vi "TestExec.Get Sequence List.vi"(8 "error in":errorcluster, 10 "Working Config File":path, 11 "Working Dir":path) -> (0 "error out":errorcluster, 1 "Default Index":i32, 2 "Sequences Info":T1[](array[typedef]), 3 "Seq Names":string[](array[string]), 4 "Repeat Delay":dbl, 6 "AutoRepeat":bool)   [LabVIEW 2018]
uses:
  Controls and Type Defs/TestExec.Sequence Info.ctl
  <vilib>/Utility/config.llb/Read Key (String).vi
  <vilib>/Utility/config.llb/Read Key (Boolean).vi
  <vilib>/Utility/config.llb/Read Key (Double).vi
  <vilib>/Utility/config.llb/NI_LVConfig.lvlib
  <vilib>/KATE/Files/File Utils.lvlib
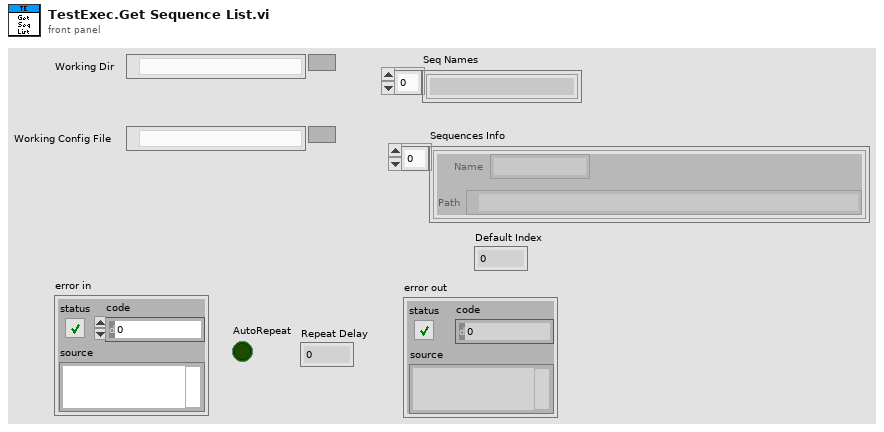
[diagram p1: front panel]
types:
  T1 = typedef "TestExec.Sequence Info.ctl" = cluster{"Name":string, "Path":path}
  T2 = typedef "NI_LVConfig.lvlib/Config Data RefNum.ctl" = refnum<k1>
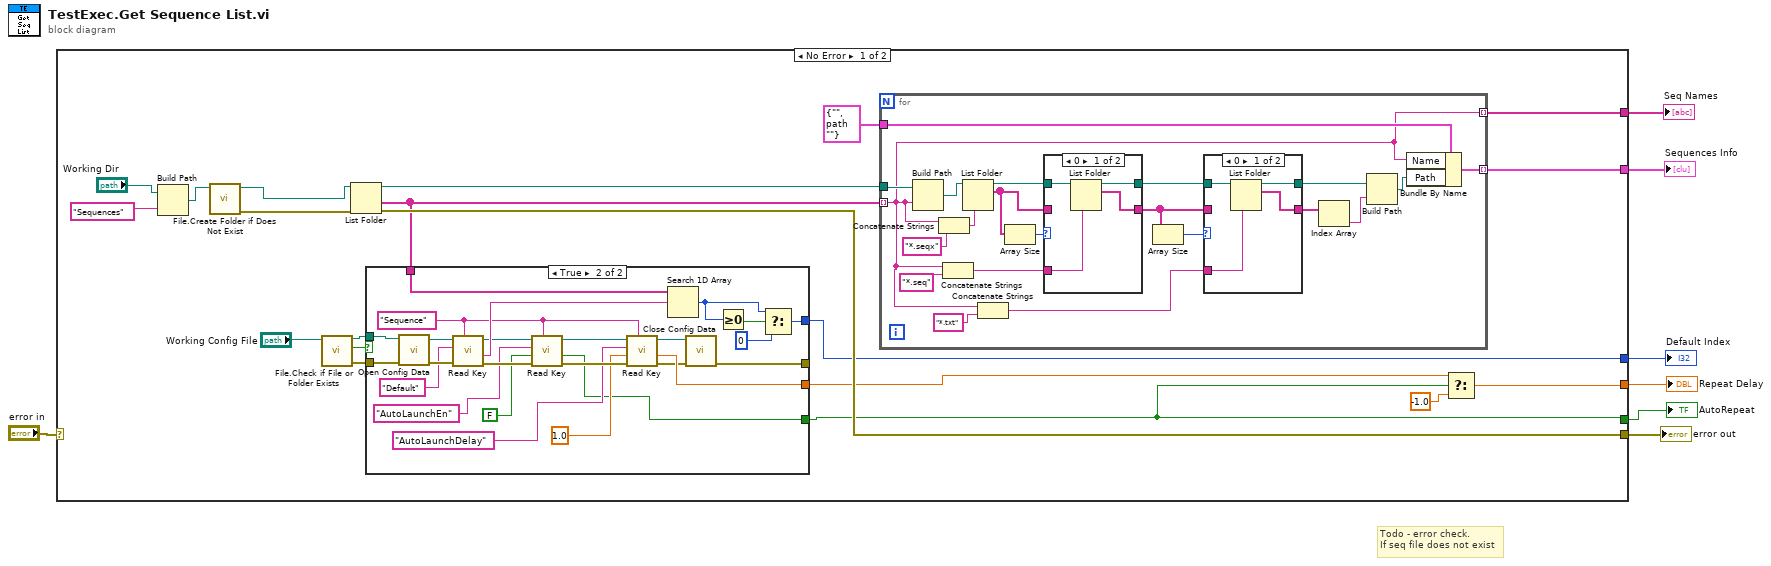
[diagram p0: block diagram]
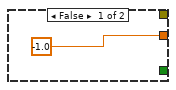
[diagram p2: hidden frame]
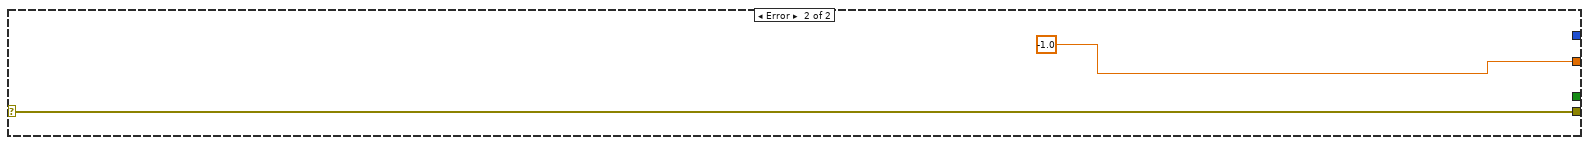
[diagram p5: hidden frame]
diagram:
  # "Todo - error check.\nIf seq file does not exist"
  n1 = case shown="No Error" "error in" {
    selector: "error in" -> [_ w88]
    tunnel: [w24 _] -> w7
    tunnel: [w23 w88] -> w5
    tunnel: [w22 _] -> w4
    tunnel: [w17 _] -> w3
    tunnel: [w12 -1.0] -> w2
    tunnel: [w9 _] -> w1
    frame No Error {
      n2 = Build Path(base path="Working Dir", name or relative path="Sequences" ("section")) -> (appended path=w16:path)
      n3 = call <vilib>:"File.Create Folder if Does Not Exist.vi"("Path"=w16) -> ("error out"=w14:errorcluster, "Dup Path"=w15:path)  [unwired: 8 in, 1 out]
      n4 = call <vilib>:"File.Check if File or Folder Exists.vi"("Path"="Working Config File") -> ("error out"=w18:errorcluster, "Exists"=w20:bool, "Dup Path"=w19:path)  [unwired: 6 in, 2 out]
      n5 = List Folder(path=w15, error in=w14) -> (path out=w26:path, folder names=w21:string[], error out=w23:errorcluster)  [unwired: 2 in, 1 out]
      n6 = case shown="True" w20 {
        tunnel: w21 -> [_ w50]
        tunnel: w19 -> [_ w49]
        tunnel: w18 -> [_ w48]
        tunnel: [_ w47] -> _
        tunnel: [_ w43] -> w17
        tunnel: [-1.0 w34] -> w11
        tunnel: [_ w29] -> w9
        frame False {
        }
        frame True {
          w35 = "Sequence"
          n7 = call <vilib>:"Open Config Data.vi"("error in (no error)"=w48, "configuration file path"=w49) -> ("error out"=w53:errorcluster, "refnum"=w52:T2)  [unwired: 7 in, 1 out]
          n8 = call-poly <vilib>:"Read Key.vi"("section"=w35, "error in (no error)"=w53, "key"="Default", "refnum"=w52) -> ("error out"=w42:errorcluster, "value"=w41:string, "refnum out"=w40:T2)  [unwired: 4 in, 1 out]
          n9 = call-poly <vilib>:"Read Key.vi"("section"=w35, "error in (no error)"=w42, "default value"=FALSE, "key"="AutoLaunchEn", "refnum"=w40) -> ("error out"=w33:errorcluster, "value"=w29:bool, "refnum out"=w37:T2)  [unwired: 3 in, 1 out]
          n10 = call-poly <vilib>:"Read Key.vi"("section"=w35, "error in (no error)"=w33, "default value"=1.0, "key"="AutoLaunchDelay", "refnum"=w37) -> ("error out"=w32:errorcluster, "value"=w34:dbl, "refnum out"=w36:T2)  [unwired: 3 in, 1 out]
          n11 = Search 1D Array(1D array=w50, element=w41) -> (index of element=w45:i32)  [unwired: 1 in]
          n12 = call <vilib>:"Close Config Data.vi"("error in (no error)"=w32, "refnum"=w36) -> ("error out"=w47:errorcluster)  [unwired: 8 in, 1 out]
          n13 = Greater Or Equal To 0?(x=w45) -> (x >= 0?=w46:bool)
          n14 = Select(t=w45, s=w46, f=0) -> (s? t:f=w43:i32)
        }
      }
      n15 = for {
        tunnel: w21 -> [w55] mode=indexing
        tunnel: w26 -> [w74]
        tunnel: T1 {"Name"="", "Path"=path ""} ("Sequence") -> [w73]
        tunnel: [w72] -> w24 mode=indexing
        tunnel: [w55] -> w22 mode=indexing
        n16 = Build Path(base path=w74, name or relative path=w55) -> (appended path=w70:path)
        n17 = Concatenate Strings(w55, "*.seqx") -> (w69:string)
        n18 = Concatenate Strings(w55, "*.seq") -> (w64:string)
        n19 = List Folder(path=w70, pattern=w69) -> (path out=w66:path, filenames=w65:string[])  [unwired: 2 in, 2 out]
        n20 = Concatenate Strings(w55, "*.txt") -> (w54:string)
        n21 = Array Size(array=w65) -> (size(s)=w67:i32)
        n22 = case shown="0" w67 {
          tunnel: w66 -> [w84 w85]
          tunnel: w65 -> [_ w86]
          tunnel: w64 -> [w81 _]
          tunnel: [w83 w86] -> w58
          tunnel: [w82 w85] -> w60
          frame 0 {
            n23 = List Folder(path=w84, pattern=w81) -> (path out=w82:path, filenames=w83:string[])  [unwired: 2 in, 2 out]
          }
          frame Default {
          }
        }
        n24 = Array Size(array=w58) -> (size(s)=w57:i32)
        n25 = case shown="0" w57 {
          tunnel: w60 -> [w78 w79]
          tunnel: w58 -> [_ w80]
          tunnel: w54 -> [w75 _]
          tunnel: [w77 w80] -> w61
          tunnel: [w76 w79] -> w59
          frame 0 {
            n26 = List Folder(path=w78, pattern=w75) -> (path out=w76:path, filenames=w77:string[])  [unwired: 2 in, 2 out]
          }
          frame Default {
          }
        }
        n27 = Index Array(array=w61) -> (element=w62:string)  [unwired: 1 in]
        n28 = Build Path(base path=w59, name or relative path=w62) -> (appended path=w63:path)
        n29 = Bundle By Name(cluster=w73, "Name"=w55, "Path"=w63) -> (w72:T1)
      }
      n30 = Select(t=w11, s=w9, f=-1.0) -> (s? t:f=w12:dbl)
    }
    frame Error {
    }
  }
  "error out" <- w5
  "Sequences Info" <- w7
  "Seq Names" <- w4
  "Default Index" <- w3
  "Repeat Delay" <- w2
  "AutoRepeat" <- w1
